vi "psmc.vi"(0 "F":dbl, 1 "H":dbl, 3 "K":dbl, 4 "L":dbl, 5 "B":dbl, 8 "pd":dbl, 9 "T":dbl, 10 "p":dbl) -> (17 "f":dbl)   [LabVIEW 2014]
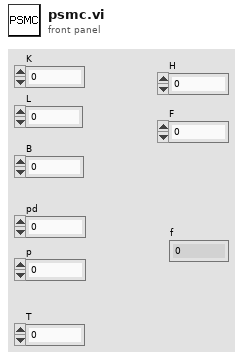
[diagram p1: front panel]
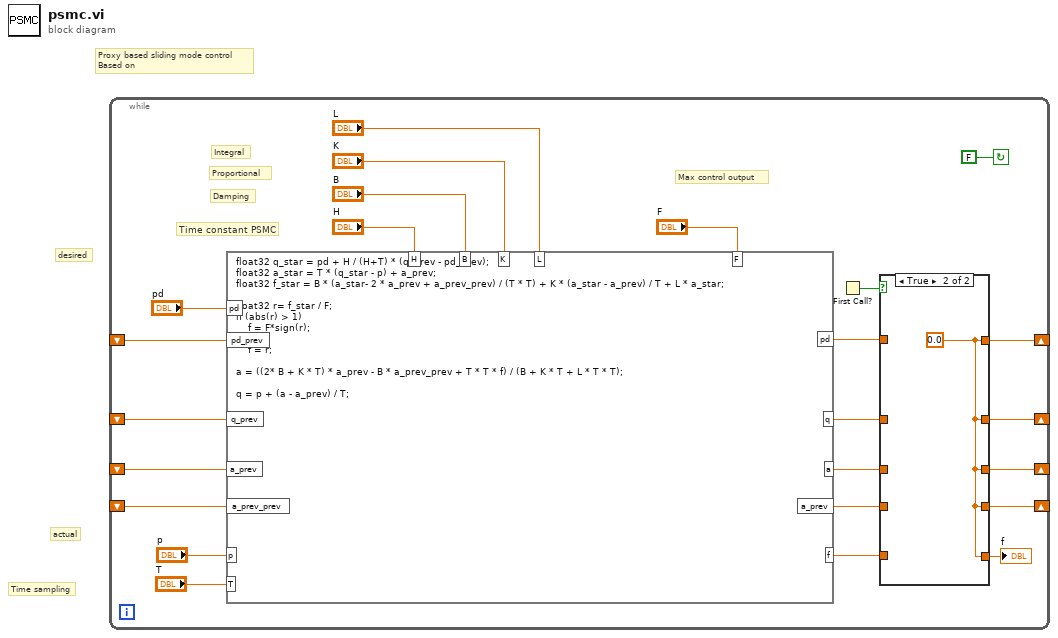
[diagram p0: block diagram]
diagram:
  # "Proxy based sliding mode control\nBased on"
  # "Time sampling"
  # "desired"
  # "actual"
  n1 = while {
    shift-right: [w20] -> _
    shift-left: _ -> [w23]
    shift-right: [w19] -> _
    shift-left: _ -> [w22]
    shift-right: [w9] -> _
    shift-left: _ -> [w7]
    shift-right: [w3] -> _
    shift-left: _ -> [w1]
    stop <- FALSE continue-if-true
    # "Max control output"
    # "Time constant PSMC"
    # "Damping"
    # "Proportional"
    # "Integral"
    n2 = formula code="float32 q_star = pd + H / (H+T) * (q_prev - pd_prev);\nfloat32 a_star = T * (q_star - p) + a_prev;\nfloat32 f_star = B * (a_star- 2 * a_prev + a_prev_prev) / (T * T) + K * (a_star - a_prev) / T + L * a_star;\n\nfloat32 r= f_star / F;\nif (abs(r) > 1)\n    f = F*sign(r);\nelse\n    f = r;\n\na = ((2* B + K * T) * a_prev - B * a_prev_prev + T * T * f) / (B + K * T + L * T * T);\n\nq = p + (a - a_prev) / T;"("T"="T", "pd_prev"=w23, "B"="B", "K"="K", "L"="L", "H"="H", "pd"="pd", "q_prev"=w22, "p"="p", "a_prev"=w7, "a_prev_prev"=w1, "F"="F") -> ("pd"=w18:dbl, "q"=w17:dbl, "a"=w8:dbl, "f"=w4:dbl, "a_prev"=w2:dbl)
    n3 = First Call?() -> (First Call?: T/F=w21:bool)
    n4 = case shown="True" w21 {
      tunnel: [w29 w30] -> w20
      tunnel: [w28 w30] -> w19
      tunnel: w18 -> [w29 _]
      tunnel: w17 -> [w28 _]
      tunnel: [w27 w30] -> w9
      tunnel: w8 -> [w27 _]
      tunnel: [w26 w30] -> w5
      tunnel: w4 -> [w26 _]
      tunnel: [w25 w30] -> w3
      tunnel: w2 -> [w25 _]
      frame False {
      }
      frame True {
        w30 = 0.0
      }
    }
    "f" <- w5
  }
